vi "main_write_summary.vi"(10 "Runtime String":refnum<vi>) -> ()   [LabVIEW 2019]
uses:
  lib/libSimulationControl/libSimulationControl.lvlib
panel:
  out "starttime - iteration":dbl
  out "sim_starttime":dbl
  out "iter":i32
  # "*******************************************************************\nBiogas Plant Control\n\nAuthor: Paul Zügel\nGCSC-Frankfurt am Main 2020\n\n*******************************************************************"
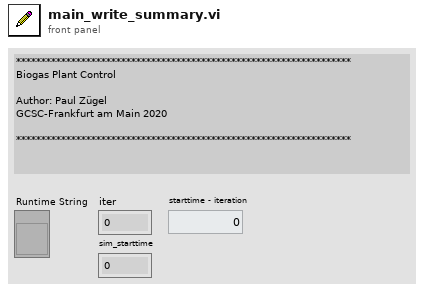
[diagram p1: front panel]
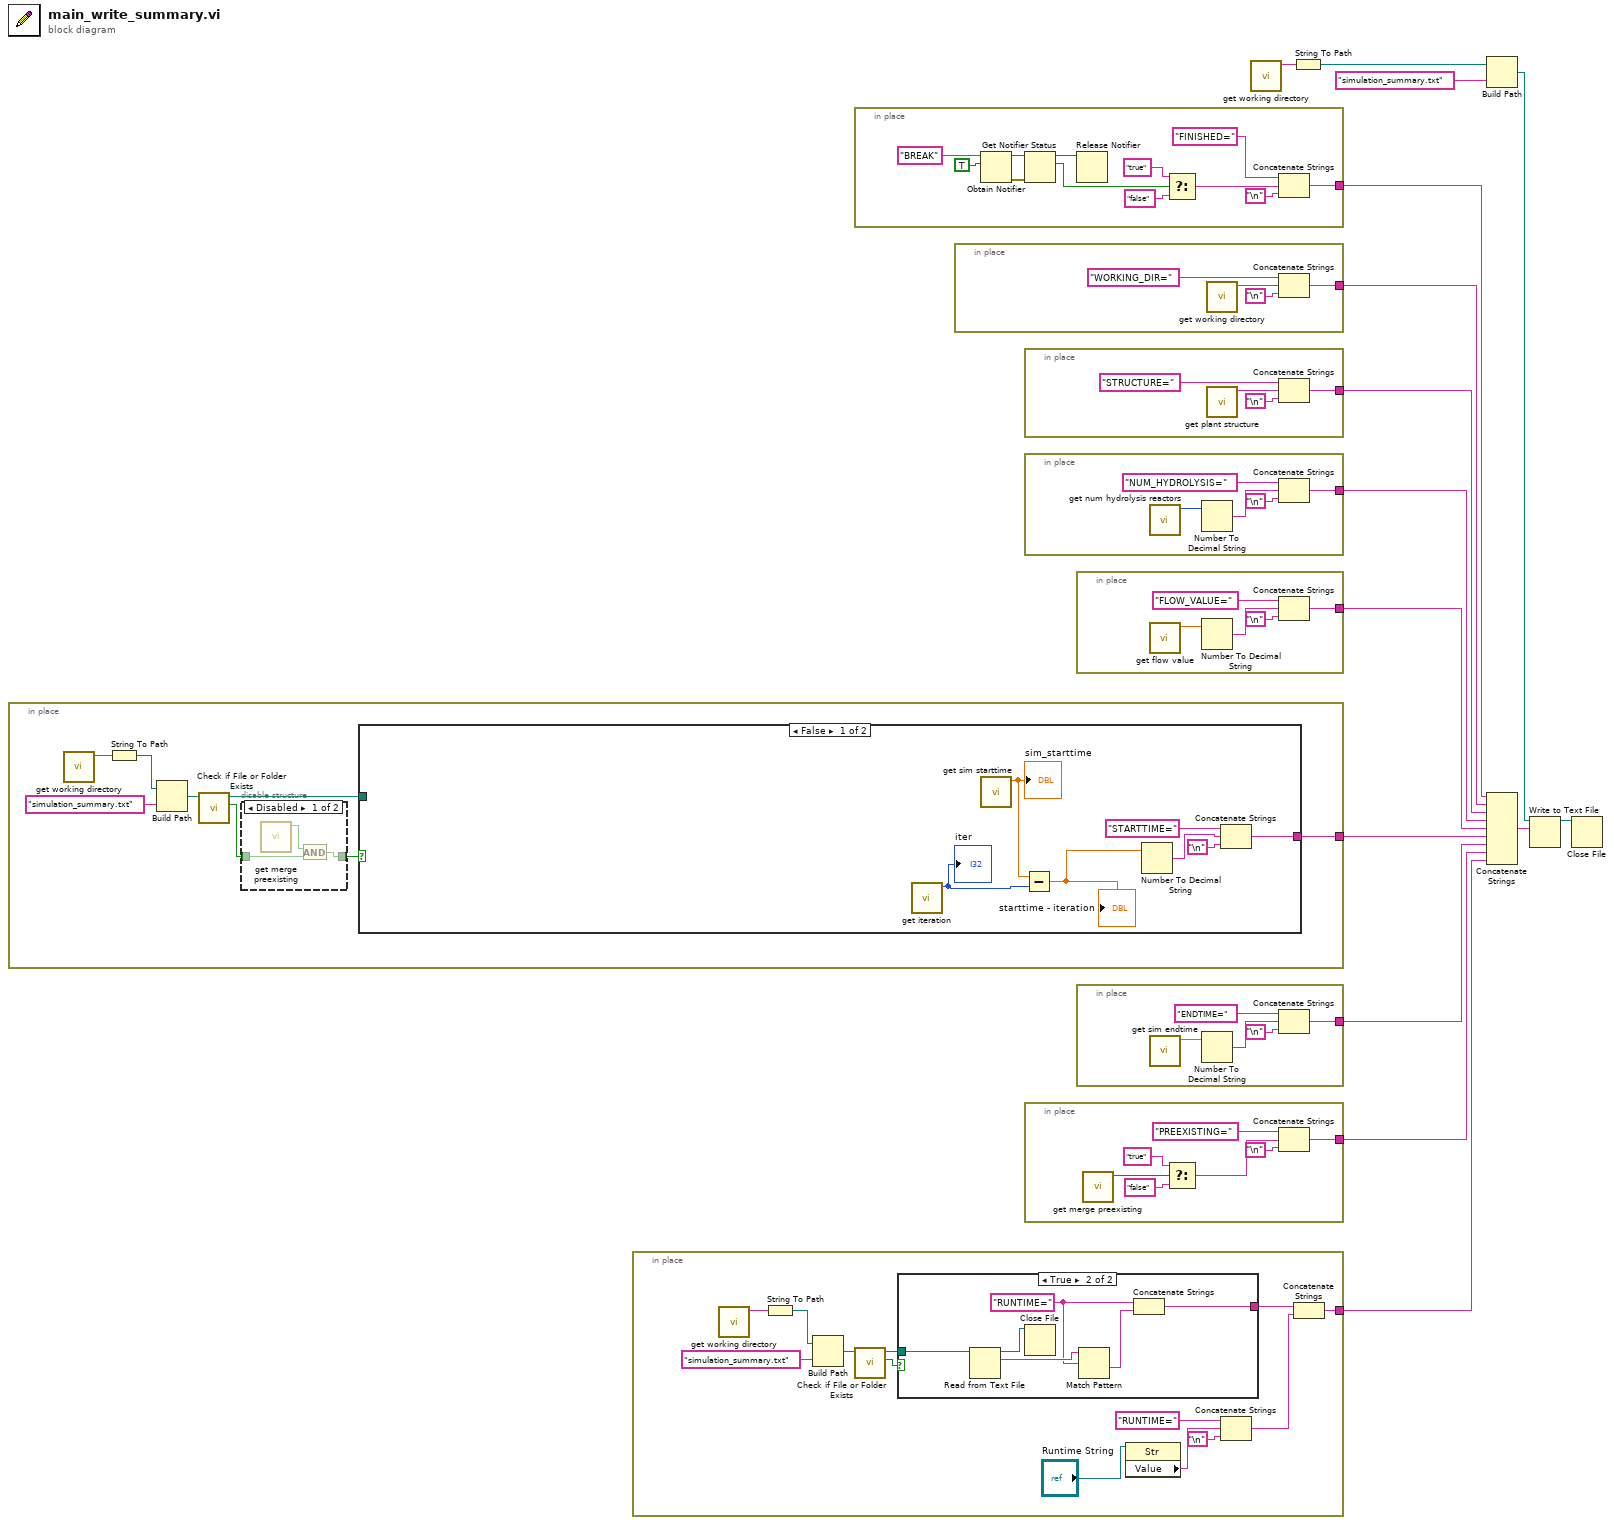
[diagram p0: block diagram]
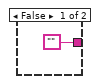
[diagram p2: hidden frame]
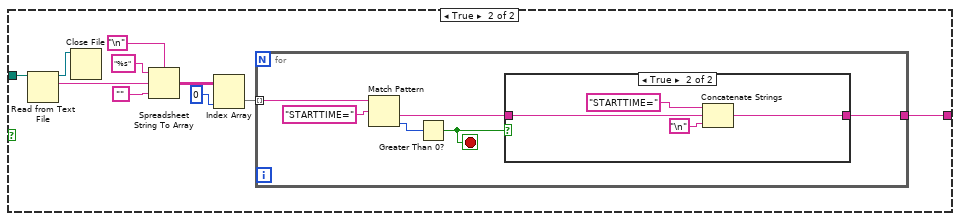
[diagram p4: hidden frame]
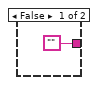
[diagram p5: hidden frame]
diagram:
  n1 = in-place {
    in-place-border: [w23] -> w4
    n2 = call "get working directory.vi"() -> ("function return"=w20:string)  [unwired: 10 in, 1 out]
    n3 = String To Path(string=w20) -> (path=w19:path)
    n4 = Build Path(base path=w19, name or relative path="simulation_summary.txt") -> (appended path=w21:path)
    n5 = call <vilib>:"Check if File or Folder Exists.vi"("path"=w21) -> ("file or folder exists?"=w22:bool, "dup path"=w16:path)  [unwired: 8 in, 1 out]
    n6 = disable-structure shown="Disabled" {
      disable-tunnel: w22 -> [w26 w27]
      disable-tunnel: [w24 w27] -> w17
      frame Disabled {
        n7 = call "get merge preexisting.vi"() -> ("function return"=w25:bool)  [unwired: 10 in, 1 out]
        n8 = And(x=w25, y=w26) -> (x .and. y?=w24:bool)
      }
      frame Enabled {
      }
    }
    n9 = case shown="False" w17 {
      tunnel: [w31 w36] -> w23
      tunnel: w16 -> [_ w44]
      frame False {
        n10 = call "get iteration.vi"() -> ("function return"=w29:i32)  [unwired: 10 in, 1 out]
        "iter" <- w29
        n11 = call "get sim starttime.vi"() -> ("sim_starttime"=w30:dbl)  [unwired: 10 in, 1 out]
        "sim_starttime" <- w30
        n12 = Subtract(x=w30, y=w29) -> (x-y=w28:dbl)
        "starttime - iteration" <- w28
        n13 = Number To Decimal String(number=w28) -> (decimal integer string=w32:string)  [unwired: 1 in]
        n14 = Concatenate Strings("STARTTIME=" ("text"), w32, "\n") -> (w31:string)
      }
      frame True {
        n15 = Read from Text File(file (use dialog)=w44) -> (refnum out=w35:refnum<file>, text=w37:string)  [unwired: 3 in, 2 out]
        n16 = Close File(refnum=w35) -> ()  [unwired: 1 in, 2 out]
        n17 = Spreadsheet String To Array(delimiter (Tab)="\n", format string="%s", spreadsheet string=w37, array type (2D Dbl)="") -> (array=w42:string[][])
        n18 = Index Array(array=w42, index (col)=0 ("disabled index (col)")) -> (element=w43:string[])  [unwired: 1 in]
        n19 = for {
          tunnel: w43 -> [w50] mode=indexing
          tunnel: [w45] -> w36
          stop <- w46 stop-if-true
          n20 = Match Pattern(string=w50, regular expression="STARTTIME=") -> (after substring=w48:string, offset past match=w49:i32)  [unwired: 1 in, 2 out]
          n21 = Greater Than 0?(x=w49) -> (x > 0?=w46:bool)
          n22 = case shown="True" w46 {
            tunnel: w48 -> [_ w53]
            tunnel: ["" w52] -> w45
            frame False {
            }
            frame True {
              n23 = Concatenate Strings("STARTTIME=" ("regular expression"), w53, "\n") -> (w52:string)
            }
          }
        }
      }
    }
  }
  n24 = in-place {
    in-place-border: [w56] -> w5
    n25 = call "get working directory.vi"() -> ("function return"=w62:string)  [unwired: 10 in, 1 out]
    n26 = String To Path(string=w62) -> (path=w63:path)
    n27 = Build Path(base path=w63, name or relative path="simulation_summary.txt") -> (appended path=w61:path)
    n28 = call <vilib>:"Check if File or Folder Exists.vi"("path"=w61) -> ("file or folder exists?"=w60:bool, "dup path"=w59:path)  [unwired: 8 in, 1 out]
    n29 = case shown="True" w60 {
      tunnel: w59 -> [_ w75]
      tunnel: ["" w71] -> w58
      frame False {
      }
      frame True {
        w72 = "RUNTIME=" ("regular expression")
        n30 = Read from Text File(file (use dialog)=w75) -> (refnum out=w70:refnum<file>, text=w74:string)  [unwired: 3 in, 2 out]
        n31 = Close File(refnum=w70) -> ()  [unwired: 1 in, 2 out]
        n32 = Match Pattern(string=w74, regular expression=w72) -> (after substring=w73:string)  [unwired: 1 in, 3 out]
        n33 = Concatenate Strings(w72, w73) -> (w71:string)
      }
    }
    n34 = property class="Str"(reference="Runtime String") -> ("Value"=w65:string)  [unwired: 1 in, 2 out]
    n35 = Concatenate Strings("RUNTIME=" ("text"), w65, "\n") -> (w57:string)
    n36 = Concatenate Strings(w58, w57) -> (w56:string)
  }
  n37 = in-place {
    in-place-border: [w77] -> w10
    n38 = Obtain Notifier(name (unnamed)="BREAK", notification data type=TRUE) -> (notifier out=w85:refnum<notifier>, error out=w84:errorcluster)  [unwired: 2 in, 1 out]
    n39 = Get Notifier Status(notifier=w85, error in (no error)=w84) -> (notifier out=w76:refnum<notifier>, current notification=w81:bool)  [unwired: 3 out]
    n40 = Release Notifier(notifier=w76) -> ()  [unwired: 2 in, 3 out]
    n41 = Select(t="true", s=w81, f="false") -> (s? t:f=w78:string)
    n42 = Concatenate Strings("FINISHED=" ("text"), w78, "\n") -> (w77:string)
  }
  n43 = in-place {
    in-place-border: [w88] -> w9
    n44 = call "get working directory.vi"() -> ("function return"=w89:string)  [unwired: 10 in, 1 out]
    n45 = Concatenate Strings("WORKING_DIR=" ("text"), w89, "\n") -> (w88:string)
  }
  n46 = in-place {
    in-place-border: [w92] -> w8
    n47 = call "get plant structure.vi"() -> ("function return"=w94:string)  [unwired: 10 in, 1 out]
    n48 = Concatenate Strings("STRUCTURE=" ("text"), w94, "\n") -> (w92:string)
  }
  n49 = in-place {
    in-place-border: [w98] -> w7
    n50 = call "get num hydrolysis reactors.vi"() -> ("function return"=w97:i32)  [unwired: 10 in, 1 out]
    n51 = Number To Decimal String(number=w97) -> (decimal integer string=w96:string)  [unwired: 1 in]
    n52 = Concatenate Strings("NUM_HYDROLYSIS=" ("text"), w96, "\n") -> (w98:string)
  }
  n53 = in-place {
    in-place-border: [w101] -> w1
    n54 = call "get merge preexisting.vi"() -> ("function return"=w105:bool)  [unwired: 10 in, 1 out]
    n55 = Select(t="true", s=w105, f="false") -> (s? t:f=w102:string)
    n56 = Concatenate Strings("PREEXISTING=" ("text"), w102, "\n") -> (w101:string)
  }
  n57 = in-place {
    in-place-border: [w110] -> w3
    n58 = call "get flow value.vi"() -> ("function return"=w108:dbl)  [unwired: 10 in, 1 out]
    n59 = Number To Decimal String(number=w108) -> (decimal integer string=w109:string)  [unwired: 1 in]
    n60 = Concatenate Strings("FLOW_VALUE=" ("text"), w109, "\n") -> (w110:string)
  }
  n61 = in-place {
    in-place-border: [w113] -> w2
    n62 = call "get sim endtime.vi"() -> ("function return"=w114:dbl)  [unwired: 10 in, 1 out]
    n63 = Number To Decimal String(number=w114) -> (decimal integer string=w115:string)  [unwired: 1 in]
    n64 = Concatenate Strings("ENDTIME=" ("text"), w115, "\n") -> (w113:string)
  }
  n65 = call "get working directory.vi"() -> ("function return"=w12:string)  [unwired: 10 in, 1 out]
  n66 = String To Path(string=w12) -> (path=w13:path)
  n67 = Build Path(base path=w13, name or relative path="simulation_summary.txt") -> (appended path=w15:path)
  n68 = Concatenate Strings(w10, w9, w8, w7, w3, w4, w2, w1, w5) -> (w11:string)
  n69 = Write to Text File(file (use dialog)=w15, text=w11) -> (refnum out=w6:refnum<file>)  [unwired: 2 in, 2 out]
  n70 = Close File(refnum=w6) -> ()  [unwired: 1 in, 2 out]
